vi "Launch Root Panel.vi"(6 "timeout in ms (-1)":i32=-1, 8 "Error In":errorcluster, 10 "Panel":refnum<class "Panel.lvclass">, 11 "Panel Actor in":refnum<class "Panel Actor.lvclass">) -> (0 "Error Out":errorcluster, 2 "Actor's Enqueuer":refnum<class "Message Enqueuer.lvclass">)   [LabVIEW 2017, in "MGI-Panel Actor.lvlib" / "Panel Actor.lvclass"]
doc: "Launches a Root Panel using any panel type.\n\n<B>Panel Actor In:</B> Panel Actor object to launch\n<B>Window Position:</B> Window Position object to control window position behavior.\n<B>timeout in ms</B> Time to wait for the panel to initialize\n<B>Error In:</B> Describes error conditions that occur before this node runs.\n\n<B>Actor's Enqueuer:</B> Enqueuer for newly spawned actor\n<B>Error Out:</B> Contains error information.\n\n----\nCopyright: MGI 2018\nAuthor: Derek Trepanier"
uses:
  Panel Actor.lvclass
  panel-manager/Source/Panel/Panel.lvclass
  <vilib>/ActorFramework/Message Enqueuer/Message Enqueuer.lvclass
  C:/Program Files (x86)/National Instruments/LabVIEW 2017/vi.lib/ActorFramework/Actor/Actor.lvclass
  panel-manager/Source/Panel/Panel.lvclass/Panel.ctl
  Panel Actor.lvclass/Panel Actor.ctl
  panel-manager/Source/Init Waiter/Init Waiter.vi
  <vilib>/ActorFramework/Actor/Actor.lvclass
  panel-manager/Source/Init Waiter/Init Waiter.lvclass
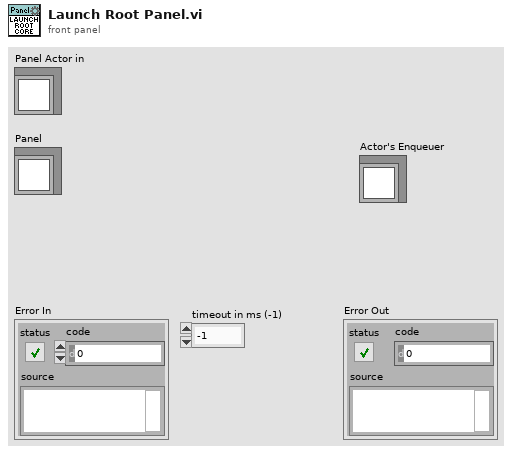
[diagram p1: front panel]
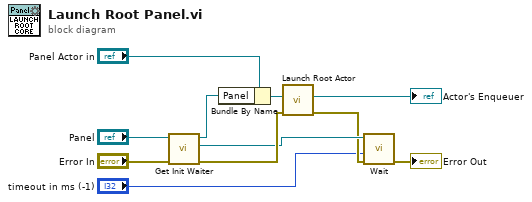
[diagram p0: block diagram]
diagram:
  n1 = call "Get Init Waiter.vi"("Error In"="Error In", "Panel In"="Panel") -> ("Error Out"=w6:errorcluster, "Init Waiter"=w5:refnum<class "Init Waiter.lvclass">, "Panel Out"=w1:refnum<class "Panel.lvclass">)  [unwired: 7 in]
  n2 = Bundle By Name(cluster="Panel Actor in", "Panel"=w1) -> (w10:refnum<class "Panel Actor.lvclass">)
  n3 = call <vilib>:"Launch Root Actor.vi"("error in (no error)"=w6, "Actor"=w10) -> ("error out"=w4:errorcluster, "Actor's Enqueuer"=→"Actor's Enqueuer":refnum<class "Message Enqueuer.lvclass">)  [unwired: 8 in]
  n4 = call "Wait.vi"("Error In"=w4, "timeout in ms (-1)"="timeout in ms (-1)", "Init Waiter in"=w5) -> ("Error Out"=→"Error Out":errorcluster)  [unwired: 6 in, 2 out]
